vi "IfTruePassConcatenated (SubVI).vi"(6 "Old Array":dbl[](array[numeric]), 9 "Loop Number":i32, 10 "Condition":dbl, 11 "New Array":dbl[](array[numeric])) -> (3 "If True, Concatenated":dbl[](array[numeric]))   [LabVIEW 2015]
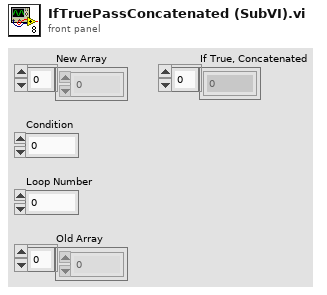
[diagram p1: front panel]
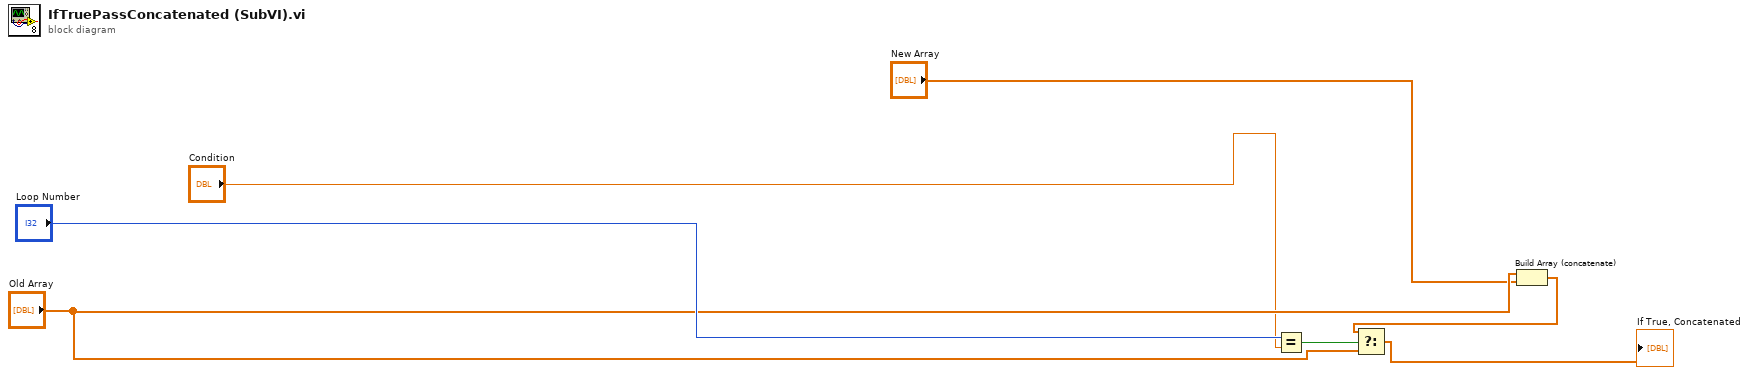
[diagram p0: block diagram]
diagram:
  n1 = Equal?(x="Loop Number", y="Condition") -> (x = y?=w1:bool)
  n2 = Build Array (concatenate)("Old Array", "New Array") -> (w2:dbl[])
  n3 = Select(t=w2, s=w1, f="Old Array") -> (s? t:f=→"If True, Concatenated":dbl[])
